vi "Read Analog Config.vi"(8 "error in (no error)":errorcluster) -> (0 "error out":errorcluster, 3 "Señal Analogica":T1={"Canal/Canales"="", "Canal"="DAQSim1", "Canales"=[], "Frecuencia de muestreo"=1000, "Numero de muestras"=1000, "Tiempo de AQ"=0.0})   [LabVIEW 2020, in "Settings.lvlib"]
uses:
  Settings.lvlib
  Aqcisition/Analog Signal Config.ctl
  <vilib>/drjdpowell/SQLite Library/SQL Connection/Open (path).vi
  <vilib>/drjdpowell/SQLite Library/SQL Connection/Open (string).vi
  <vilib>/AdvancedString/Path To Command Line String.vi
  <vilib>/drjdpowell/SQLite Library/SQL Connection/Execute SQL (1D String).vi
  <vilib>/drjdpowell/SQLite Library/SQL Connection/Connection.lvclass
  <vilib>/drjdpowell/SQLite Library/SQLite.lvlib
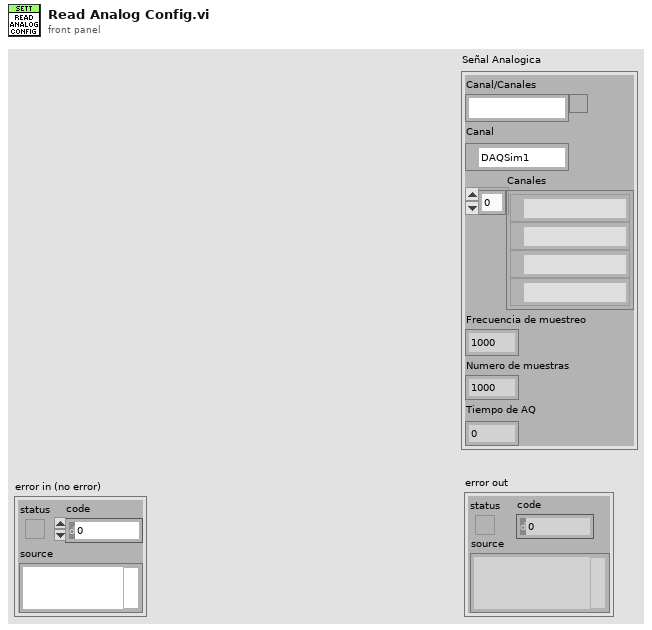
[diagram p1: front panel]
types:
  T1 = typedef "Analog Signal Config.ctl" = cluster{"Canal/Canales":string, "Canal":tag, "Canales":tag[], "Frecuencia de muestreo":i32, "Numero de muestras":i32, "Tiempo de AQ":dbl}
  T2 = cluster{"Text":string, "Text":string, "Text":string, "Text":string}
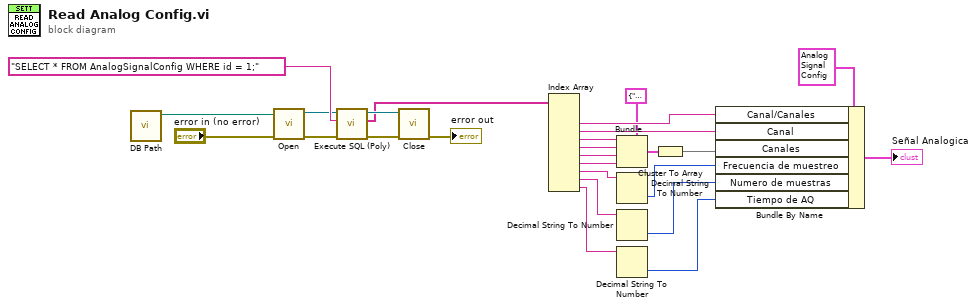
[diagram p0: block diagram]
diagram:
  n1 = call "DB Path.vi"() -> ("appended path"=w18:path)  [unwired: 11 in]
  n2 = call-poly <vilib>:"Open.vi"("error in (no error)"="error in (no error)", "db file"=w18) -> ("error out"=w26:errorcluster, "SQLite Connection"=w21:refnum<class "Connection.lvclass">)  [unwired: 8 in]
  n3 = call-poly <vilib>:"Execute SQL (Poly).vi"("error in (no error)"=w26, "SQL"="SELECT * FROM AnalogSignalConfig WHERE id = 1;", "SQLite Connection in"=w21) -> ("error out"=w25:errorcluster, "Result Set"=w19:string[], "SQLite Connection"=w20:refnum<class "Connection.lvclass">)  [unwired: 5 in, 1 out]
  n4 = call-dynamic "Close.vi"("error in (no error)"=w25, "SQLite Connection in"=w20) -> ("error out"=→"error out":errorcluster)  [unwired: 9 in]
  n5 = Index Array(array=w19) -> (element #2=w15:string, element #3=w14:string, element #4=w13:string, element #5=w12:string, element #6=w11:string, element #7=w10:string, element #8=w6:string, element #9=w5:string, element #10=w4:string)  [unwired: 10 in, 1 out]
  n6 = Bundle(cluster=T2 {"Text"="", "Text"="", "Text"="", "Text"=""}, "Text"=w13, "Text"=w12, "Text"=w11, "Text"=w10) -> (w8:T2)
  n7 = Decimal String To Number(string=w6) -> (number=w3:i32)  [unwired: 2 in, 1 out]
  n8 = Decimal String To Number(string=w5) -> (number=w2:i32)  [unwired: 2 in, 1 out]
  n9 = Decimal String To Number(string=w4) -> (number=w1:i32)  [unwired: 2 in, 1 out]
  n10 = Cluster To Array(cluster=w8) -> (array=w7:string[])
  n11 = Bundle By Name(cluster=T1 {"Canal/Canales"="", "Canal"="DAQSim1", "Canales"=[], "Frecuencia de muestreo"=1000, "Numero de muestras"=1000, "Tiempo de AQ"=0.0} ("Señal Analogica"), "Canal/Canales"=w15, "Canal"=w14, "Canales"=w7, "Frecuencia de muestreo"=w3, "Numero de muestras"=w2, "Tiempo de AQ"=w1) -> (→"Señal Analogica":T1)
